vi "APLUS Camille Bauer Driver.vi"(8 "error in (no error)":errorcluster, 9 "Reset WattHours":bool, 10 "Remote Port":u16=502, 11 "Remote IP Address":string="192.168.1.101") -> (0 "error out":errorcluster, 2 "Power":sgl, 3 "Power Data":T1={"Current (A):Element 1"=236.2, "Current (A):Element 2"=17.749, "Power (W):Sigma"=4192.0, "Watt Hours (Wh):Sigma"=0.0, "Voltage (V):Element 2"=236.2, "Voltage (V):Element 1"=236.2, "Current Crest Factor:Element 1"=0.0, "Current Crest Factor:Element 2"=0.0, "Voltage Harmonic (%):Element 1"=0.0, "Voltage Harmonic (%):Element 2"=0.0, "Voltage Crest Factor:Element 1"=0.0, "Voltage Crest Factor:Element 2"=0.0, "Time:Element 1"=0.0, "Frequency (Hz):Element 1"=0.0, "Apparent Power (VA):Element 1"=0.0, "Apparent Power (VA):Element 2"=0.0, "Power Factor:Element 1"=0.0, "Power Factor:Element 2"=0.0, "Max Watt Hours"=0.0, "Voltage (V):Element 2 Avg"=0.0, "Voltage (V):Element 1 Avg"=0.0} {"Voltage (V):Element 1 Avg" format="%.3g"; "Voltage (V):Element 2 Avg" format="%.3g"; "Max Watt Hours" format="%.3g"; "Power Factor:Element 2" format="%.3g"; "Power Factor:Element 1" format="%.3g"; "Apparent Power (VA):Element 2" format="%.3g"; "Apparent Power (VA):Element 1" format="%.3g"; "Frequency (Hz):Element 1" format="%.3g"; "Time:Element 1" format="%.3g"; "Voltage Crest Factor:Element 2" format="%.3g"; "Voltage Crest Factor:Element 1" format="%.3g"; "Voltage Harmonic (%):Element 2" format="%.3g"; "Voltage Harmonic (%):Element 1" format="%.3g"; "Current Crest Factor:Element 2" format="%.3g"; "Current Crest Factor:Element 1" format="%.3g"; "Voltage (V):Element 1" format="%.3g"; "Voltage (V):Element 2" format="%.3g"; "Watt Hours (Wh):Sigma" format="%.3f"; "Power (W):Sigma" format="%.3g"; "Current (A):Element 2" format="%.3e"; "Current (A):Element 1" format="%.3e"}, 5 "APLUS Data":string[][](array[string]), 7 "APLUS DBL Data":dbl[](array[numeric]))   [LabVIEW 2019]
uses:
  Trunk/Utility/Type Definitions/UTILITY Power Data.ctl
  <vilib>/NI/Modbus Library/API/Wrapper/Create TCP Master.vi
  <vilib>/NI/Modbus Library/API/Master/Modbus Master.lvclass
  <vilib>/NI/Modbus Library/API/Wrapper/API Main.lvlib
panel:
  out "Watt Hours (kWh)":dbl
  # "TCP Parameters"
  # "Data to write to the slave"
  # "Slave Read-only Registers"
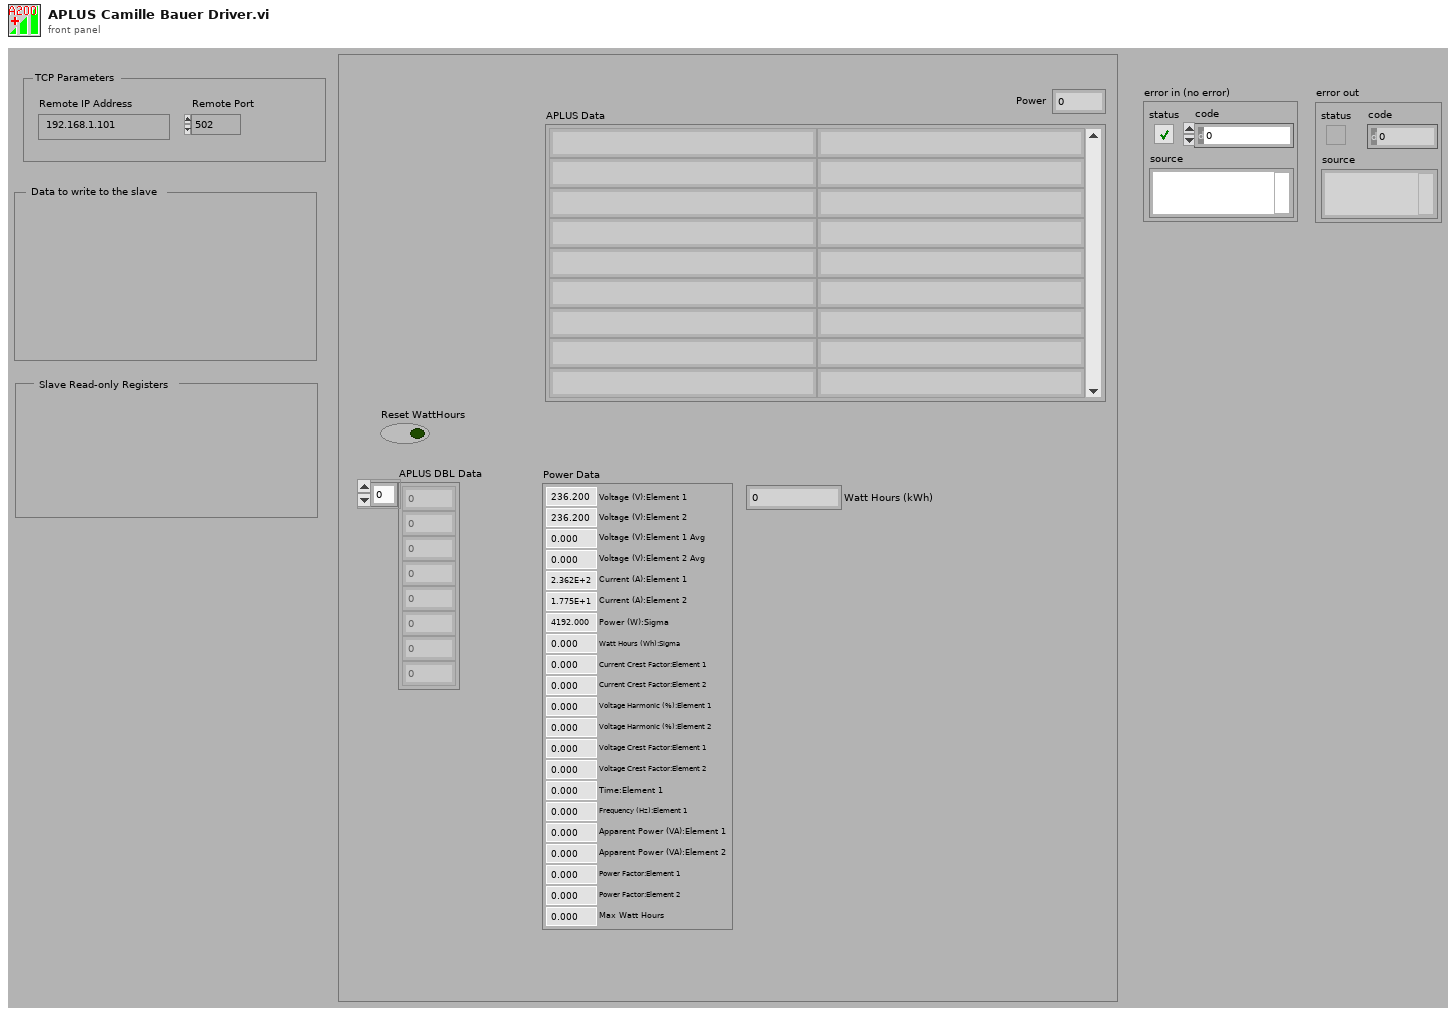
[diagram p1: front panel]
types:
  T1 = typedef "UTILITY Power Data.ctl" = cluster{"Current (A):Element 1":dbl, "Current (A):Element 2":dbl, "Power (W):Sigma":dbl, "Watt Hours (Wh):Sigma":dbl, "Voltage (V):Element 2":dbl, "Voltage (V):Element 1":dbl, "Current Crest Factor:Element 1":dbl, "Current Crest Factor:Element 2":dbl, "Voltage Harmonic (%):Element 1":dbl, "Voltage Harmonic (%):Element 2":dbl, "Voltage Crest Factor:Element 1":dbl, "Voltage Crest Factor:Element 2":dbl, "Time:Element 1":dbl, "Frequency (Hz):Element 1":dbl, "Apparent Power (VA):Element 1":dbl, "Apparent Power (VA):Element 2":dbl, "Power Factor:Element 1":dbl, "Power Factor:Element 2":dbl, "Max Watt Hours":dbl, "Voltage (V):Element 2 Avg":dbl, "Voltage (V):Element 1 Avg":dbl}
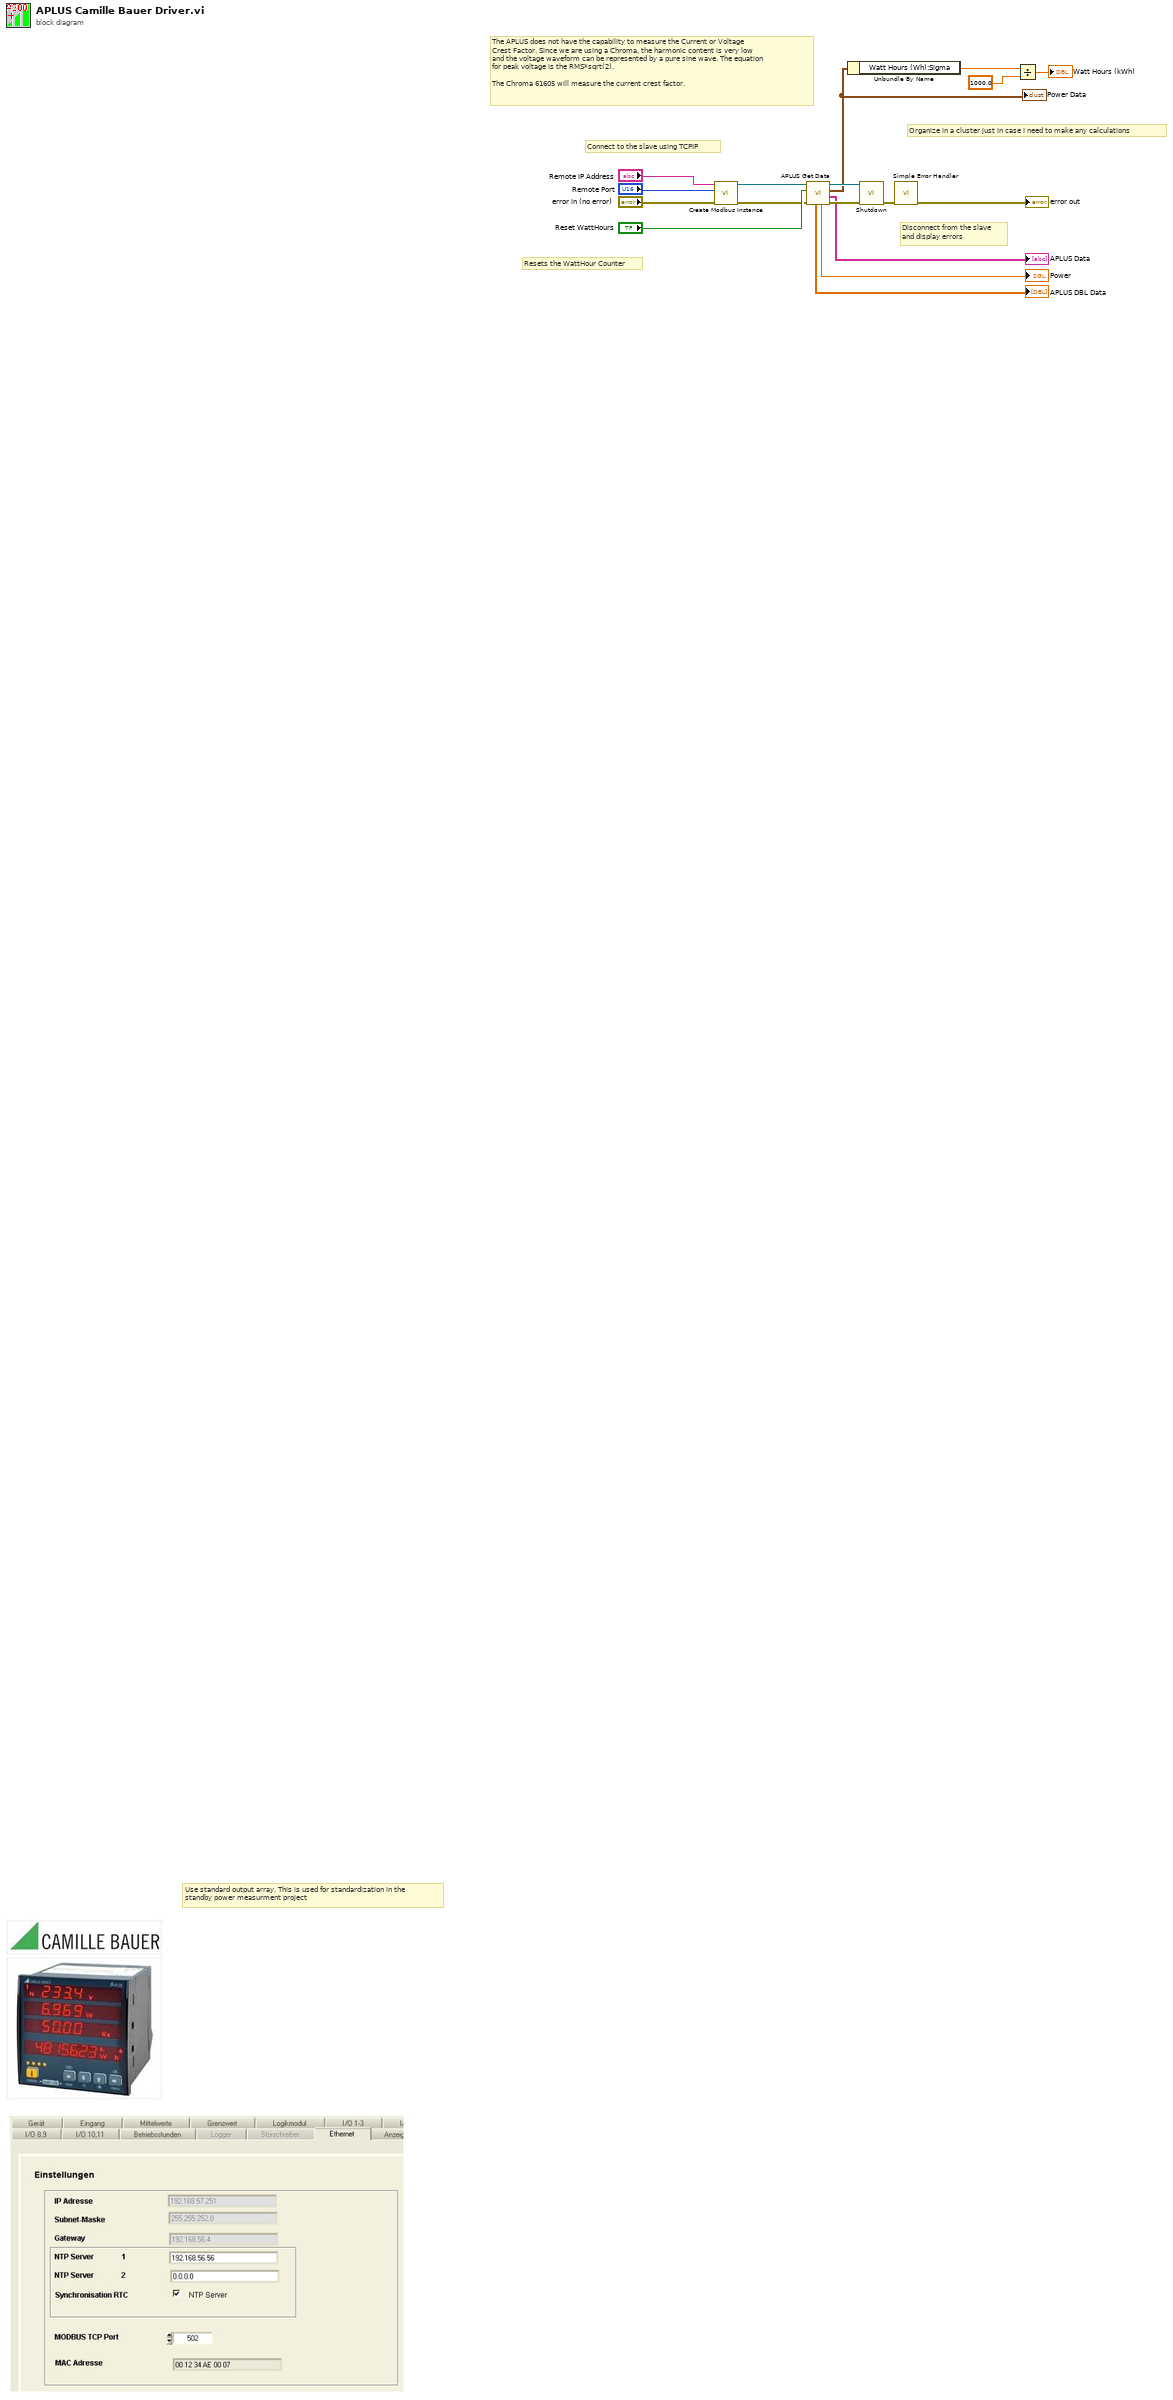
[diagram p0: block diagram]
diagram:
  # "Organize in a cluster just in case I need to make any calculations"
  # "Use standard output array. This is used for standardization in the \nstandby power measurment project"
  # "The APLUS does not have the capability to measure the Current or Voltage \nCrest Factor. Since we are using a Chroma, the harmonic content is very low\nand the voltage waveform can be represented by a pure sine wave. The equation\nfor peak voltage is the RMS*sqrt(2). \n\nThe Chroma 61605 will measure the current crest factor."
  # "Resets the WattHour Counter"
  # "Disconnect from the slave\nand display errors"
  # "Connect to the slave using TCPIP"
  n1 = call-poly <vilib>:"Create Modbus Instance.vi"("error in"="error in (no error)", "port (502)"="Remote Port", "address"="Remote IP Address") -> ("error out"=w12:errorcluster, "TCP master instance"=w8:refnum<class "Modbus Master.lvclass">)  [unwired: 7 in]
  n2 = call "APLUS Get Data.vi"("error in (no error)"=w12, "Reset WattHours"="Reset WattHours", "Modbus Master in"=w8) -> ("error out"=w13:errorcluster, "APLUS Data"=→"APLUS Data":string[][], "PowerData"=w5:T1, "Modbus Master out"=w14:refnum<class "Modbus Master.lvclass">, "Power"=→"Power":sgl, "APLUS DBL Data"=→"APLUS DBL Data":dbl[])  [unwired: 3 in]
  "Power Data" <- w5
  n3 = Unbundle By Name(w5) -> ("Watt Hours (Wh):Sigma"=w4:dbl)
  n4 = call-dynamic "Shutdown.vi"("error in"=w13, "Modbus master in"=w14) -> ("error out"=w16:errorcluster)  [unwired: 9 in]
  n5 = call <vilib>:"Simple Error Handler.vi"("error in (no error)"=w16) -> ("error out"=→"error out":errorcluster)  [unwired: 1 in, 7 out]
  n6 = Divide(x=w4, y=1000.0) -> (x/y=→"Watt Hours (kWh)":dbl)
